vi "SHA-512-256.vi"() -> (0 "Hash Function out":refnum<class "NI_SHA-512.lvclass">)   [LabVIEW 2020, in "NI_SHA-512.lvclass"]
doc: "Returns an instance of the SHA-512/256 hash function."
uses:
  <vilib>/security/Message Digest/SHA-2/SHA-512/NI_SHA-512.lvclass
  <vilib>/security/Message Digest/SHA-2/SHA-512/subVIs/Mode.ctl
  <vilib>/security/Message Digest/SHA-2/SHA-512/NI_SHA-512.lvclass/NI_SHA-512.ctl
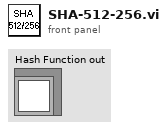
[diagram p1: front panel]
types:
  T1 = typedef "NI_SHA-512.lvclass/Mode.ctl" = enum16{"SHA-512", "SHA-384", "SHA-512/256", "SHA-512/224"}
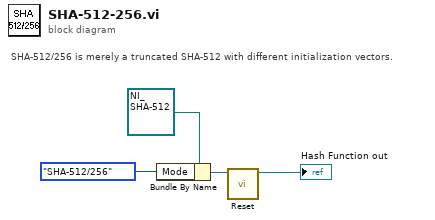
[diagram p0: block diagram]
diagram:
  # "SHA-512/256 is merely a truncated SHA-512 with different initialization vectors."
  n1 = Bundle By Name(cluster=refnum<class "NI_SHA-512.lvclass"> refnum ("nihash-sha2.lvlib:SHA-512.lvclass"), "Mode"=Mode."SHA-512/256") -> (w2:refnum<class "NI_SHA-512.lvclass">)
  n2 = call <vilib>:"Reset.vi"("Hash Function in"=w2) -> ("Hash Function out"=→"Hash Function out":refnum<class "NI_SHA-512.lvclass">)  [unwired: 10 in]
